vi "DataStream_RT_Close.vi"(8 "Error":errorcluster, 11 "Stream Ref":T1) -> (0 "Error Out":errorcluster)   [LabVIEW 2020]
uses:
  <vilib>/ErrorRing/Error Ring.xnode
  TypeDefs/Cluster_DataStream_RT Writer Refs.ctl
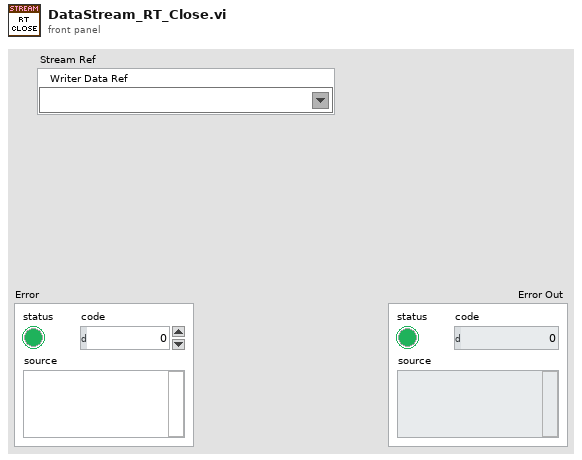
[diagram p1: front panel]
types:
  T1 = typedef "Cluster_DataStream_RT Writer Refs.ctl" = cluster{"Writer Data Ref":refnum<k21>}
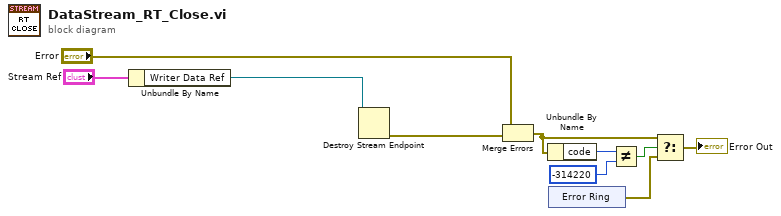
[diagram p0: block diagram]
diagram:
  n1 = Unbundle By Name("Stream Ref") -> ("Writer Data Ref"=w4:refnum<k21>)
  n2 = Destroy Stream Endpoint(11:w4) -> (0:w2:errorcluster)  [unwired: 1 in]
  n3 = Merge Errors("Error", w2) -> (w3:errorcluster)
  n4 = Unbundle By Name(w3) -> ("code"=w6:i32)
  n5 = xnode "Error Ring"() -> ("error out"=w9:errorcluster)
  n6 = Not Equal?(x=w6, y=-314220) -> (x != y?=w8:bool)
  n7 = Select(t=w3, s=w8, f=w9) -> (s? t:f=→"Error Out":errorcluster)
